vi "WaitOn_Queue.vi"(6 "Tag Root":string, 8 "Max Queue Size":i32=-1, 9 "Timeout (ms)":i32=-1, 10 "Message Type":variant, 11 "Queue Name":string) -> (0 "error out":errorcluster, 2 "Omni Bus Out":refnum<class "Omni_Bus.lvclass">, 3 "Queue out":refnum<class "bt_WaitOn_Queue.lvclass">)   [LabVIEW 2021, in "BT.lvlib"]
uses:
  BT.lvlib
  <vilib>/TSA/Omni-Bus/Omni-Bus/Omni_Bus.lvclass
  Support/Nodes/Leaves/Synch/Queue/WaitOn/bt_WaitOn_Queue.lvclass
  C:/Users/Tim/Documents/GitHub/LV_Behaviour_Tree/Source/Support/Nodes/Leaves/Synch/Parent/WaitOn/bt_WaitOn_Synch.lvclass
  <vilib>/TSA/Omni-Bus/Aggregator Bus/Aggregator Bus.lvclass
  C:/Program Files (x86)/National Instruments/LabVIEW 2021/vi.lib/TSA/Omni-Bus/Omni-Bus/Bus Access/Bus_Access.lvclass
  Support/Nodes/Leaves/Synch/Queue/WaitOn/bt_WaitOn_Queue.lvclass/bt_WaitOn_Queue.ctl
  Support/Nodes/Leaves/Synch/Parent/WaitOn/bt_WaitOn_Synch.lvclass/bt_WaitOn_Synch.ctl
  Support/Nodes/Leaves/Synch/Queue/WaitOn/Properties/Write Initialise Error.vi
  Support/Nodes/Leaves/Synch/Queue/WaitOn/Properties/Write Omni Bus.vi
  Support/Nodes/Leaves/Synch/Queue/WaitOn/Properties/Write Value Objects.vi
  Support/Nodes/Leaves/Synch/Queue/WaitOn/Properties/Write types.vi
  Support/Nodes/Leaves/Synch/Queue/WaitOn/Properties/Write Name.vi
  Support/Nodes/Leaves/Synch/Queue/WaitOn/Properties/Write Max Queue Size.vi
  Support/Nodes/Leaves/Synch/Parent/WaitOn/Properties/Write Timeout.vi
  <vilib>/TSA/Abstract Data Classes/Abs_Types/Value/Abs_Value.lvclass
  C:/Program Files (x86)/National Instruments/LabVIEW 2021/vi.lib/TSA/Abstract Data Classes/Abs_Types/Type/Abs_Type.lvclass
  Support/Nodes/Leaves/Synch/With Values/WaitOn/bt_WaitOn_Synch_WithValues.lvclass
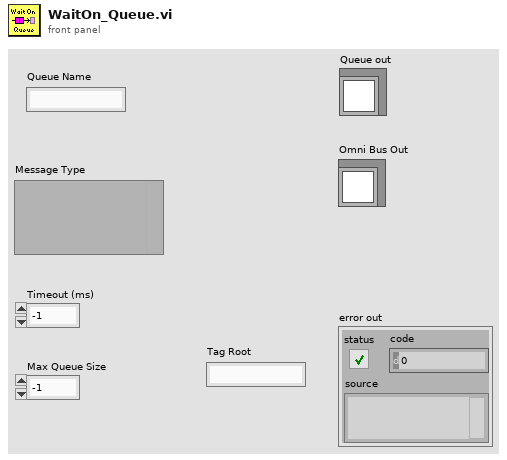
[diagram p1: front panel]
types:
  T1 = typedef "NI_Data Type.lvlib/Data Type.ctl" = enum8{"Invalid Type", "Void", "I8", "I16", "I32", "I64", "U8", "U16", "U32", "U64", "Single Float", "Double Float", "Extended Float", "Single Complex", "Double Complex", "Extended Complex", "Enum U8", "Enum U16", "Enum U32", "Enum U64", "Single Float With Unit", "Double Float With Unit", "Extended Float With Unit", "Single Complex with Unit", "Double Complex with Unit", "Extended Complex with Unit", "Boolean", "String", "Path", "Picture", "Tag", "Array", "Cluster", "Variant", "LV Variant", "Waveform", "Timestamp", "Digital Waveform", "Digital Data", "ExpressData", "Refnum", "External Data", "VI", "Poly VI", "LabVIEW Class Instance", "Fixed Point", "Set Collection", "Map Collection"}
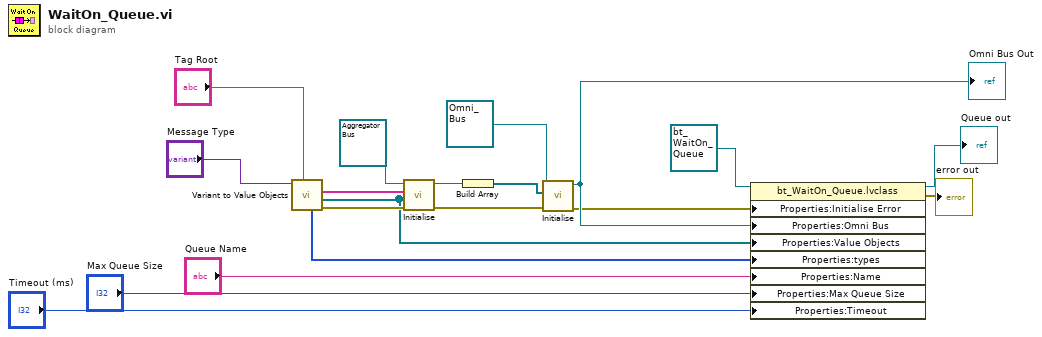
[diagram p0: block diagram]
diagram:
  n1 = call "Variant to Value Objects.vi"("Name Root"="Tag Root", "Variant"="Message Type") -> ("error out"=w17:errorcluster, "Value Objects OUT"=w8:refnum<class "Abs_Value.lvclass">[], "Names OUT"=w18:string[], "types out"=w7:T1[])  [unwired: 6 in]
  n2 = call <vilib>:"Initialise.vi"("error in (no error)"=w17, "Values"=w8, "Tags"=w18, "Aggregator Bus in"=refnum<class "Aggregator Bus.lvclass"> refnum) -> ("error out"=w11:errorcluster, "Aggregator Bus out"=w14:refnum<class "Aggregator Bus.lvclass">)  [unwired: 6 in]
  n3 = Build Array(w14) -> (w13:refnum<class "Aggregator Bus.lvclass">[])
  n4 = call-dynamic <vilib>:"Initialise.vi"("error in (no error)"=w11, "Bus Access"=w13, "Var Bus in"=refnum<class "Omni_Bus.lvclass"> refnum) -> ("error out"=w2:errorcluster, "Var Bus out"=w9:refnum<class "Omni_Bus.lvclass">)  [unwired: 7 in]
  "Omni Bus Out" <- w9
  n5 = property class="bt_WaitOn_Queue.lvclass"(reference=refnum<class "bt_WaitOn_Queue.lvclass"> refnum ("BT.lvlib:bt_WaitOn_Queue.lvclass"), "Properties:Initialise Error"=w2, "Properties:Omni Bus"=w9, "Properties:Value Objects"=w8, "Properties:types"=w7, "Properties:Name"="Queue Name", "Properties:Max Queue Size"="Max Queue Size", "Properties:Timeout"="Timeout (ms)") -> (reference out=→"Queue out":refnum<class "bt_WaitOn_Queue.lvclass">, error out=→"error out":errorcluster)  [unwired: 1 in]
